vi "DataVIS_Differentiate_and_Rebundle_inPlace.vi"(7 "Fit Points":dbl, 8 "error in (no error)":errorcluster, 11 "Data Cell In":T1(array[cluster])) -> (0 "error out":errorcluster, 3 "Data Cell":T1(array[cluster]))   [LabVIEW 2016]
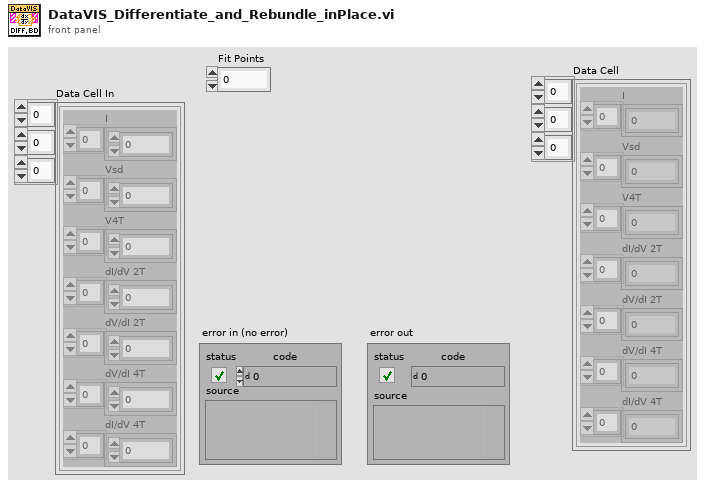
[diagram p1: front panel]
types:
  T1 = cluster{"I":dbl[], "Vsd":dbl[], "V4T":dbl[], "dI/dV 2T":dbl[], "dV/dI 2T":dbl[], "dV/dI 4T":dbl[], "dI/dV 4T":dbl[]}[][][]
  T2 = cluster{"I":dbl[], "Vsd":dbl[], "V4T":dbl[], "dI/dV 2T":dbl[], "dV/dI 2T":dbl[], "dV/dI 4T":dbl[], "dI/dV 4T":dbl[]}
  T3 = cluster{"Decimated Array":dbl[], "Decimated Array":dbl[]}
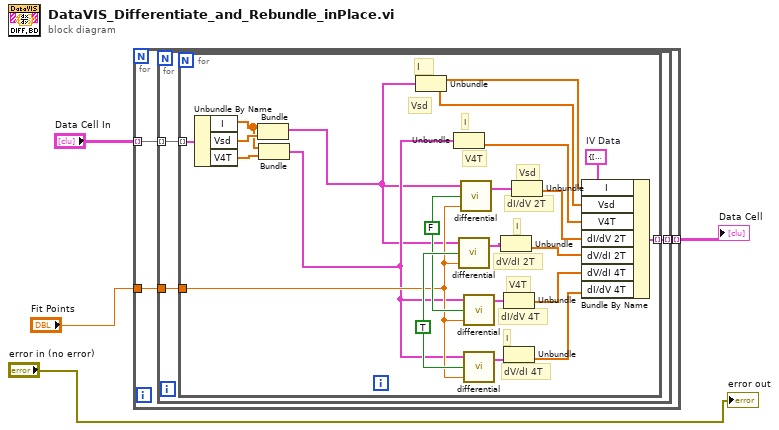
[diagram p0: block diagram]
diagram:
  n1 = for {
    tunnel: [w7] -> w3 mode=indexing
    tunnel: "Fit Points" -> [w6]
    tunnel: "Data Cell In" -> [w5] mode=indexing
    n2 = for {
      tunnel: [w10] -> w7 mode=indexing
      tunnel: w6 -> [w9]
      tunnel: w5 -> [w8] mode=indexing
      n3 = for {
        tunnel: [w18] -> w10 mode=indexing
        tunnel: w9 -> [w17]
        tunnel: w8 -> [w16] mode=indexing
        w26 = T2 {"I"=[], "Vsd"=[], "V4T"=[], "dI/dV 2T"=[], "dV/dI 2T"=[], "dV/dI 4T"=[], "dI/dV 4T"=[]}  # IV Data
        w31 = FALSE ("dy/dx vs x")
        w32 = TRUE ("dy/dx vs x")
        # "V4T"
        # "I"
        # "Vsd"
        # "I"
        # "dV/dI 4T"
        # "I"
        # "dI/dV 4T"
        # "V4T"
        # "dV/dI 2T"
        # "I"
        # "dI/dV 2T"
        # "Vsd"
        n4 = Unbundle By Name(w16) -> ("I"=w14:dbl[], "Vsd"=w15:dbl[], "V4T"=w13:dbl[])
        n5 = Bundle("I"=w14, "Vsd"=w15) -> (w11:cluster{"I":dbl[], "Vsd":dbl[]})  [unwired: 1 in]
        n6 = Bundle("I"=w14, "V4T"=w13) -> (w12:cluster{"I":dbl[], "V4T":dbl[]})  [unwired: 1 in]
        n7 = Unbundle(w11) -> ("I"=w25:dbl[], "Vsd"=w24:dbl[])
        n8 = Unbundle(w12) -> ("V4T"=w23:dbl[])  [unwired: 1 out]
        n9 = call <userlib>:"differential.vi"("Numeric"=w17, "dy/dx vs x"=w32, "A vs B 2"=w11) -> ("A vs B 3"=w27:T3)  [unwired: 1 in]
        n10 = call <userlib>:"differential.vi"("Numeric"=w17, "dy/dx vs x"=w31, "A vs B 2"=w11) -> ("A vs B 3"=w30:T3)  [unwired: 1 in]
        n11 = call <userlib>:"differential.vi"("Numeric"=w17, "dy/dx vs x"=w31, "A vs B 2"=w12) -> ("A vs B 3"=w28:T3)  [unwired: 1 in]
        n12 = call <userlib>:"differential.vi"("Numeric"=w17, "dy/dx vs x"=w32, "A vs B 2"=w12) -> ("A vs B 3"=w29:T3)  [unwired: 1 in]
        n13 = Unbundle(w27) -> ("Decimated Array"=w21:dbl[])  [unwired: 1 out]
        n14 = Unbundle(w28) -> ("Decimated Array"=w20:dbl[])  [unwired: 1 out]
        n15 = Unbundle(w29) -> ("Decimated Array"=w19:dbl[])  [unwired: 1 out]
        n16 = Unbundle(w30) -> ("Decimated Array"=w22:dbl[])  [unwired: 1 out]
        n17 = Bundle By Name(cluster=w26, "I"=w25, "Vsd"=w24, "V4T"=w23, "dI/dV 2T"=w22, "dV/dI 2T"=w21, "dV/dI 4T"=w20, "dI/dV 4T"=w19) -> (w18:T2)
      }
    }
  }
  "Data Cell" <- w3
  "error out" <- "error in (no error)"
